vi "InitializeCamAndTF.vi"(8 "Camera":i32, 10 "Path to keras folder":path) -> (0 "error out":errorcluster, 3 "TFinfo out":T1)   [LabVIEW 2019]
panel:
  out "resulting string":string
  out "Numeric":u8
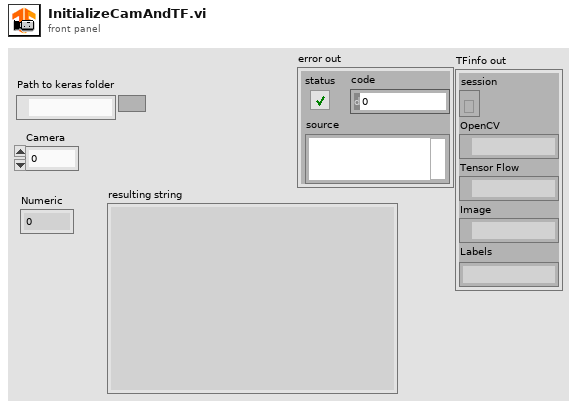
[diagram p1: front panel]
types:
  T1 = cluster{"session":refnum<k35>, "OpenCV":path, "Tensor Flow":path, "Image":path, "Labels":string}
  T2 = cluster{"session out":refnum<k35>, "appended path":path, "appended path":path, "appended path":path, string}
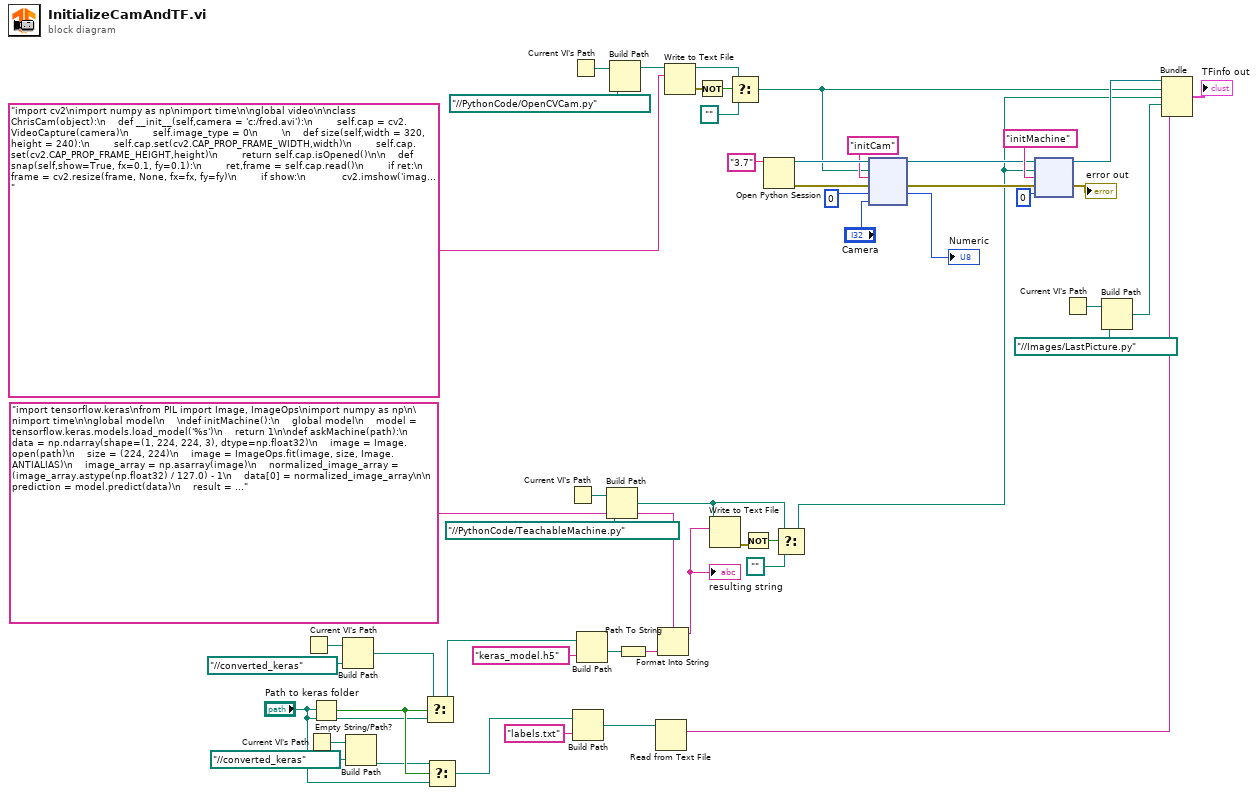
[diagram p0: block diagram]
diagram:
  n1 = Current VI's Path() -> (path=w18:path)
  n2 = Current VI's Path() -> (path=w14:path)
  n3 = Empty String/Path?(string/path="Path to keras folder") -> (empty?=w7:bool)
  n4 = Build Path(base path=w18, name or relative path=path "../../converted_keras") -> (appended path=w11:path)
  n5 = Build Path(base path=w14, name or relative path=path "../../converted_keras") -> (appended path=w6:path)
  n6 = Select(t=w11, s=w7, f="Path to keras folder") -> (s? t:f=w10:path)
  n7 = Select(t=w6, s=w7, f="Path to keras folder") -> (s? t:f=w4:path)
  n8 = Current VI's Path() -> (path=w29:path)
  n9 = Current VI's Path() -> (path=w31:path)
  n10 = Build Path(base path=w4, name or relative path="labels.txt") -> (appended path=w2:path)
  n11 = Build Path(base path=w10, name or relative path="keras_model.h5") -> (appended path=w8:path)
  n12 = Build Path(base path=w29, name or relative path=path "../../PythonCode/TeachableMachine.py") -> (appended path=w27:path)
  n13 = Build Path(base path=w31, name or relative path=path "../../PythonCode/OpenCVCam.py") -> (appended path=w43:path)
  n14 = Path To String(path=w8) -> (string=w16:string)
  n15 = Read from Text File(file (use dialog)=w2) -> (text=w12:string)  [unwired: 3 in, 3 out]
  n16 = Format Into String(format string="import tensorflow.keras\nfrom PIL import Image, ImageOps\nimport numpy as np\n\nimport time\n\nglobal model\n    \ndef initMachine():\n    global model\n    model = tensorflow.keras.models.load_model('%s')\n    return 1\n\ndef askMachine(path):\n    data = np.ndarray(shape=(1, 224, 224, 3), dtype=np.float32)\n    image = Image.open(path)\n    size = (224, 224)\n    image = ImageOps.fit(image, size, Image.ANTIALIAS)\n    image_array = np.asarray(image)\n    normalized_image_array = (image_array.astype(np.float32) / 127.0) - 1\n    data[0] = normalized_image_array\n\n    prediction = model.predict(data)\n    result = prediction.tolist()\n    return result\n" ("name or relative path"), w16) -> (resulting string=w15:string)  [unwired: 2 in, 1 out]
  "resulting string" <- w15
  n17 = Write to Text File(file (use dialog)=w43, text="import cv2\nimport numpy as np\nimport time\n\nglobal video\n\nclass ChrisCam(object):\n    def __init__(self,camera = 'c:/fred.avi'):\n        self.cap = cv2.VideoCapture(camera)\n        self.image_type = 0\n        \n    def size(self,width = 320, height = 240):\n        self.cap.set(cv2.CAP_PROP_FRAME_WIDTH,width)\n        self.cap.set(cv2.CAP_PROP_FRAME_HEIGHT,height)\n        return self.cap.isOpened()\n\n    def snap(self,show=True, fx=0.1, fy=0.1):\n        ret,frame = self.cap.read()\n        if ret:\n            frame = cv2.resize(frame, None, fx=fx, fy=fy)\n        if show:\n            cv2.imshow('image',frame)\n        return ret, frame\n\n    def rotate(self, img, rotation):\n        rows,cols,depth = img.shape\n        rotationMatrix = cv2.getRotationMatrix2D((cols/2,rows/2),rotation,1)\n        frame = cv2.warpAffine(img,rotationMatrix,(cols,rows))\n        return frame\n\n    def toLV(self,frame,plane = 'RGB'):      # takes around 30 ms per call\n        array = frame.ravel()\n        mask = np.array([])\n        if not plane == 'Gray':\n            image_depth = 24\n            colors = np.array([])\n            fixedFrame = np.empty((array.size,),dtype = array.dtype)\n            if 'R' in plane:\n                fixedFrame[0::3] = array[2::3]   # go from BGR ro RGB\n            if 'G' in plane:\n                fixedFrame[1::3] = array[1::3]\n            if 'B' in plane:\n                fixedFrame[2::3] = array[0::3]\n        else:\n            fixedFrame = np.empty((int(array.size/3),),dtype = array.dtype)\n            fixedFrame[0::1] = array[0::3]# int((int(array[0::3]) + int(array[1::3]) +  int(array[2::3]) ) / 3)\n            image_depth = 8\n            colors = np.array([ (i | i<<8 | i<<16) for i in range(256)])  # define color map\n        self.rectangle = (0,0,frame.shape[1],frame.shape[0])  # this is the LabVIEW rectangle format\n        reply =  (self.image_type, image_depth,fixedFrame.tolist(),mask.tolist(),colors.tolist(),self.rectangle)\n        return reply\n\n    def toCV(self,LVimage):      # takes around 30 ms per call\n        rows,cols = LVimage[5][3],LVimage[5][2]\n        array = np.asarray(LVimage[2],dtype='uint8')\n        fixedFrame = np.empty((array.size,),dtype = array.dtype)\n        fixedFrame[0::3] = array[2::3]   # go from RGB to BGR\n        fixedFrame[1::3] = array[1::3]\n        fixedFrame[2::3] = array[0::3]\n        img = fixedFrame.reshape(rows,cols,3)\n        return img\n\n    def close(self):\n        self.cap.release()\n        cv2.destroyAllWindows()\n        return True\n\ndef initCam(camera = 'c:/fred.avi',width = 640, height = 480):\n    global video\n    video = ChrisCam(camera)\n    return video.size(width,height)\n\ndef snap(show=True, rotation = 90, plane = 'RGB',fx=0.1, fy=0.1):\n    ret, frame = video.snap(show,fx,fy)\n    if not ret:\n        return \n    if not rotation == 0:\n        frame = video.rotate(frame,rotation)\n    return video.toLV(frame,plane)\n\ndef closeCam():\n    return video.close()\n\n") -> (error out=w40:errorcluster)  [unwired: 2 in, 2 out]
  n18 = Not(x=w40) -> (.not. x?=w41:bool)
  n19 = Write to Text File(file (use dialog)=w27, text=w15) -> (error out=w49:errorcluster)  [unwired: 2 in, 2 out]
  n20 = Select(t=w43, s=w41, f=path "") -> (s? t:f=w25:path)
  n21 = Not(x=w49) -> (.not. x?=w47:bool)
  n22 = Open Python Session(python version="3.7" ("Python version")) -> (session out=w46:refnum<k35>, error out=w39:errorcluster)  [unwired: 2 in]
  n23 = Select(t=w27, s=w47, f=path "") -> (s? t:f=w24:path)
  n24 = node(w46, w25, "initCam" ("function name"), w39, u8 0, "Camera") -> (w32:refnum<k35>, w34:errorcluster, →"Numeric":u8)  [unwired: 1 in, 2 out]
  n25 = node(w32, w24, "initMachine" ("function name"), w34, u8 0) -> (w26:refnum<k35>, →"error out":errorcluster)  [unwired: 1 in, 2 out]
  n26 = Current VI's Path() -> (path=w22:path)
  n27 = Build Path(base path=w22, name or relative path=path "../../Images/LastPicture.py") -> (appended path=w20:path)
  n28 = Bundle("session out"=w26, "appended path"=w25, "appended path"=w24, "appended path"=w20, w12) -> (→"TFinfo out":T2)  [unwired: 1 in]
